vi "Waveform Creation.vi"(8 "Amplitude":dbl, 9 "Max sample rate":dbl, 10 "Frequency":dbl, 11 "Cant. Freq":dbl) -> (1 "Samples":i32, 3 "Waveform Graph":waveform(dbl)(graph))   [LabVIEW 2018]
panel:
  out "dt":dbl
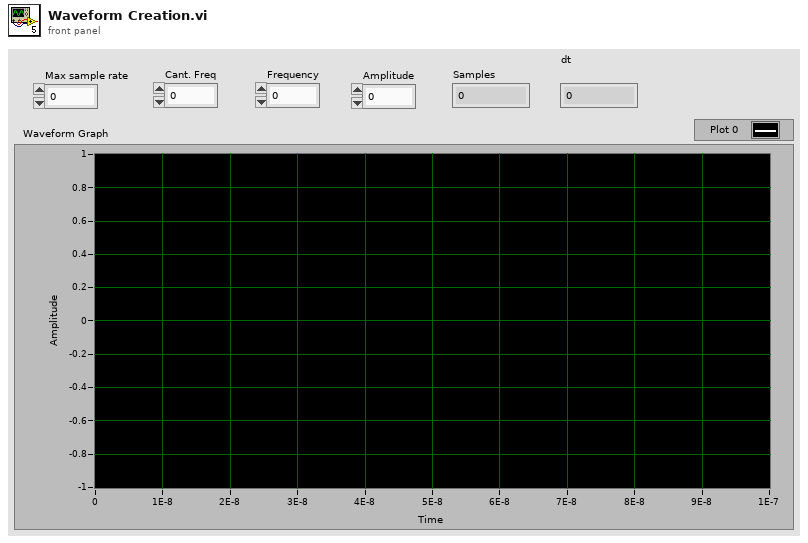
[diagram p1: front panel]
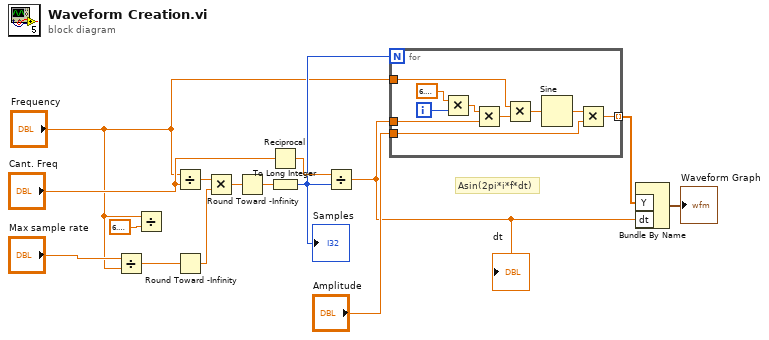
[diagram p0: block diagram]
diagram:
  # "Asin(2pi*i*f*dt)"
  n1 = Divide(x="Max sample rate", y="Frequency") -> (x/y=w5:dbl)
  n2 = Divide(x="Frequency", y=6.283185307179586) -> ()  [unwired: 1 out]
  n3 = Divide(x="Frequency", y="Cant. Freq") -> (x/y=w11:dbl)
  n4 = Round Toward -Infinity(1:w5) -> (0:w4:dbl)
  n5 = Multiply(x=w11, y=w4) -> (x*y=w10:dbl)
  n6 = Round Toward -Infinity(1:w10) -> (0:w3:dbl)
  n7 = Reciprocal(x="Cant. Freq") -> (1/x=w7:dbl)
  n8 = To Long Integer(number=w3) -> (32bit integer=w2:i32)
  "Samples" <- w2
  n9 = Divide(x=w7, y=w2) -> (x/y=w6:dbl)
  "dt" <- w6
  n10 = for {
    N: w2 -> [_]
    tunnel: [w17] -> w15 mode=indexing
    tunnel: "Frequency" -> [w21]
    tunnel: "Amplitude" -> [w19]
    tunnel: w6 -> [w16]
    i -> [w24]
    n11 = Multiply(x=6.283185307179586, y=w24) -> (x*y=w23:dbl)
    n12 = Multiply(x=w23, y=w16) -> (x*y=w20:dbl)
    n13 = Multiply(x=w21, y=w20) -> (x*y=w22:dbl)
    n14 = Sine(x=w22) -> (sin(x)=w18:dbl)
    n15 = Multiply(x=w18, y=w19) -> (x*y=w17:dbl)
  }
  n16 = Bundle By Name("Y"=w15, "dt"=w6) -> (→"Waveform Graph":waveform(dbl))  [unwired: 1 in]
